vi "根据点击位置找索引.vi"(1 "坐标":cluster{"水平":i32, "垂直":i32}, 2 "位置":cluster{"左":i32, "顶":i32}, 3 "边界":cluster{"高":i32, "宽":i32}) -> (0 "索引":i32)   [LabVIEW 2017]
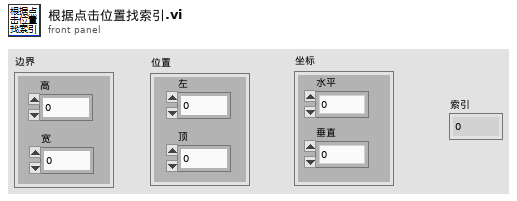
[diagram p1: front panel]
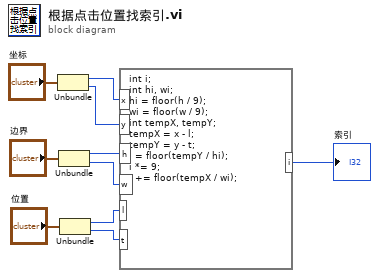
[diagram p0: block diagram]
diagram:
  n1 = Unbundle("坐标") -> ("水平"=w7:i32, "垂直"=w6:i32)
  n2 = Unbundle("边界") -> ("高"=w5:i32, "宽"=w4:i32)
  n3 = Unbundle("位置") -> ("左"=w3:i32, "顶"=w2:i32)
  n4 = formula code="int i;\nint hi, wi;\nhi = floor(h / 9);\nwi = floor(w / 9);\nint tempX, tempY;\ntempX = x - l;\ntempY = y - t;\ni = floor(tempY / hi);\ni *= 9;\ni += floor(tempX / wi);"("x"=w7, "y"=w6, "l"=w3, "t"=w2, "h"=w5, "w"=w4) -> ("i"=→"索引":i32)
